vi "FetchRX.vi"(8 "error in (no error)":errorcluster, 11 "reference in":refnum<class "niMmWave_Reciever.lvclass">) -> (0 "error out":errorcluster, 2 "RX burst data":refnum<class "mmWave data.lvclass">, 3 "reference out":refnum<class "niMmWave_Reciever.lvclass">)   [LabVIEW 2019, in "niMmWave_Reciever.lvclass"]
doc: "Fetches RX IQ data from isnturment"
uses:
  niMmWave_Reciever.lvclass
  C:/Barkhausen mmWave radar/Development/modules/mmw_instrument/src_LabVIEW/Host/SubVIs/mmWave instrument_class/mmWave instrument.lvclass
  mmWave data_class/mmWave data.lvclass
  mmWave HW Control/HW custom error.ctl
  mmWave instrument_class/Instrument state.ctl
  IQBurst_memo_class/IQBurst_memo.lvclass
  C:/Barkhausen mmWave radar/Development/modules/mmw_instrument/src_LabVIEW/Host/SubVIs/mmWave data_class/mmWave data.lvclass
  23a7541f-384f-44a9-b270-a12c5ae2c0ad.vi
  <vilib>/addons/Modulation/Analog/MT Resample (Complex Cluster).vi
  <vilib>/addons/Modulation/Analog/support/Validators/mod_Fractional Resample Validate.vi
  <vilib>/addons/Modulation/Analog/support/Validators/mod_Check Flush State.vi
  <vilib>/addons/Modulation/Analog/support/mod_FractionalResampler.vi
  <vilib>/addons/Modulation/Analog/support/mod_Integer Rate Interpolation.vi
  <vilib>/addons/Modulation/Analog/support/mod_Set Error Source.vi
  <vilib>/addons/Modulation/Analog/support/Validators/mod_Validate Complex Waveform.vi
  <vilib>/addons/Modulation/Analog/support/mod_PerformResampling.vi
  <vilib>/addons/Modulation/Analog/support/Validators/mod_WFErrorHandler.vi
  <userlib>/_OpenG.lib/string/string.llb/Trim Whitespace (String)__ogtk.vi
  <vilib>/Utility/error.llb/Error Cluster From Error Code.vi
  <vilib>/addons/Modulation/Analog/support/mod_Resampling Factors.vi
  <vilib>/addons/Modulation/Analog/support/mod_ResamplingFilter.vi
  <vilib>/addons/Modulation/Analog/support/mod_Generate Integer Interpolation Filter.vi
  mmWave HW Control/mmWave HW Control.lvlib
  mmWave instrument_class/mmWave instrument.lvclass
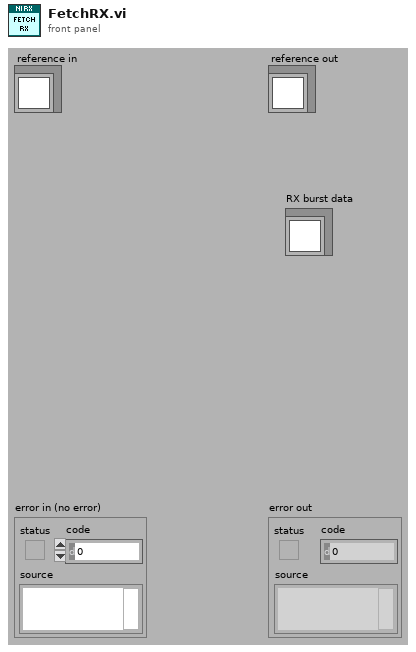
[diagram p1: front panel]
types:
  T1 = typedef "mmWave instrument.lvclass/Instrument state.ctl" = enum16{"Off", "Initialization", "Configuration", "Running", "Calibration"}
  T2 = typedef "mmWave HW Control.lvlib/HW custom error.ctl" = u16
  T3 = typedef "niMmWave_Reciever.lvclass/ObjectAttributesRef.ctl" = refnum<data-value>
  T4 = typedef "niMmWave_Reciever.lvclass/ObjectAttributes.ctl" = cluster{"session":T5[], "HW.RX devices":T19, "RF config":T20, "RX trigger options":T21, "RX samples":i32, "RX Fs":dbl}
  T5 = typedef "Session.ctl" = cluster{"3620 session":refnum<queue>, "tx baseband session":T6, "rx baseband session":T14, "tx gain (dB)":dbl, "rx gain (dB)":dbl, "hardware configuration":T15, "gain ranging":T17[], "pxi trigger bus information":T18}
  T6 = typedef "Tx Baseband Session.ctl" = cluster{"3610 session":T7, "7902 reference":T13}
  T7 = typedef "ni3610_and_ni3630_Driver_Lib.lvlib/Main Settings.ctl" = cluster{"VISA resource name":refnum<visa-resource-name>, "Address Space":T8, "window_offset":u32, "register_addresses":T9, "required_MM_fpga_version":cluster{"signature":u32, "hardware":u32, "current revision":u32, "oldest revision":u32}, "CPLD Oldest Compat Version ":cluster{"hardware":u32, "CPLD firmware":u32}, "MM_FPGA_image_location":string, "is_init":bool, "card_type":T10, "DacLmkConfigFileName":string, "AdcLmkConfigFileName":string, "AdcConfigFileName":string, "DacConfigFileName_RevA":string, "DacConfigFileName_RevB":string, "Mulde hardware revision":u8, "bypass DAC PLL\n":bool, "IQ Card Revision":T11, "board capability":T12}
  T8 = typedef "VISA Register Access Address Space.ctl" = u16
  T9 = typedef "ni3610_and_ni3630_Driver_Lib.lvlib/Register Adresses.ctl" = cluster{"MM based Registers":cluster{"Revision":u32, "OldestCompatRev":u32, "signature":u32, "scratch":u32, "LedControl":u32, "BoardHwRev":u32, "BoardControl":u32, "ThermalStatus":u32, "BasebandStatus":u32, "BasebandControl":u32, "BasebandAuxSetup":u32, "BasebandAuxStatus":u32, "LmkSyncOutSetup":u32, " AdcSyncOutSetup":u32, " InjSyncOutSetup":u32, " PxiTrig0OutSetup":u32, " PxiTrig1OutSetup":u32, " PxiTrig2OutSetup":u32, " PxiTrig3OutSetup":u32, " PxiTrig4OutSetup":u32, " PxiTrig5OutSetup":u32, " PxiTrig6OutSetup":u32, " PxiTrig7OutSetup":u32}, "CPLD based Registers":cluster{"SlaveSignature":u32, "SlaveRevision":u32, "SlaveOldestCompatRev":u32, "SlaveScratch":u32, "SlaveSetup":u32, "SlaveStatus":u32, "IDacReg_offset":u32, "LMKRegGrp0_offset":u32, "QDacReg_offset":u32, "BrdTempSensorVal":u32, "TempSensorPowerDown":u32, "GPIOReg_offset":u32, "IAdcReg_offset":u32, "QAdcReg_offset":u32, "LMKRegGrp1_offset":u32, "QadcTempSensorVal":u32, "IadcTempSensorVal":u32, "RevisionReg":u32, "VcxoReg":u32, "CpldStatusReg":u32, "PowerReg":u32, "VBiasEnReg":u32, "ExtRefOeReg":u32, "QdacCtrlReg":u32, "QdacStatusReg":u32, "IdacCtrlReg":u32, "IdacStatusReg":u32, "QdacJtagIn":u32, "QdacJtagOut":u32, "IdacJtagIn":u32, "IdacJtagOut":u32, "IqDcSetupReg":u32, "QadcStatusReg":u32, "IadcStatusReg":u32, "BrdSetupReg":u32, "IqDcRevisionReg":u32, "PllStatusReg":u32, "EndpointScratchReg":u32, "AdcSyncCfgReg":u32, "IqCardOpampReg":u32}, "CPLD Register Offset":u32, "MM  Register Offset":u32, " PxiTrig0OutSetup":u32}
  T10 = typedef "ni3610_and_ni3630_Driver_Lib.lvlib/Base Card Type.ctl" = enum16{"unspecified", "ADC", "DAC"}
  T11 = typedef "ni3610_and_ni3630_Driver_Lib.lvlib/IQ Card Revision.ctl" = enum16{"RevA", "RevB", "RevC", "RevD"}
  T12 = typedef "ni3610_and_ni3630_Driver_Lib.lvlib/Board Capability.ctl" = cluster{"baseband sync":enum16{"no baseband sync", "baseband sync"}}
  T13 = typedef "Blank FPGA Reference.ctl" = refnum<k20>
  T14 = typedef "Rx Baseband Session.ctl" = cluster{"3630 session":T7, "7902 reference":T13}
  T15 = typedef "Hardware Configuration.ctl" = cluster{"direction":T16, "baseband only":bool}
  T16 = typedef "Direction.ctl" = enum16{"Transceiver", "Receiver", "Transmitter"}
  T17 = typedef "Gain Ranging.ctl" = cluster{"gain ranging active scope":string, "gain ranging stream session":refnum<k20>}
  T18 = typedef "PXI Trigger Bus Info.ctl" = cluster{"chassis resource name":refnum<visa-resource-name>, "7902R (TX)":i16, "3610 (TX)":i16, "3620 (IF)":i16, "3630 (RX)":i16, "7902R (RX)":i16}
  T19 = typedef "mmWave HW Control.lvlib/HW RX resources cluster.ctl" = cluster{"HW.IF":tag, "HW.ADC":refnum<visa-resource-name>, "HW.RX FPGA":tag}
  T20 = typedef "mmWave HW Control.lvlib/HW RX RF config cluster.ctl" = cluster{"Gain":dbl, "Frequency":dbl, "mmWave adapter":string}
  T21 = typedef "TX trigger config.ctl" = cluster{"delay":dbl, "trig source":T22, "PXI src":i32, "export":T23, "PXI dest":i32}
  T22 = typedef "FPGA Utility.lvlib/FPGA driver trigger source.ctl" = enum16{"Use Tclk", "PXI_Trig", "Aurora RX trig"}
  T23 = typedef "FPGA Utility.lvlib/FPGA driver trigger destination.ctl" = enum16{"None", "Source trig", "Synced trig", "Delayed sync"}
  T24 = typedef "Constants.ctl" = cluster{"data clock rate (Hz)":dbl, "sample rate (Hz)":dbl, "sample rate selector string":string, "default tx bitfile path":path, "default rx bitfile path":path, "default proc bitfile path":path}
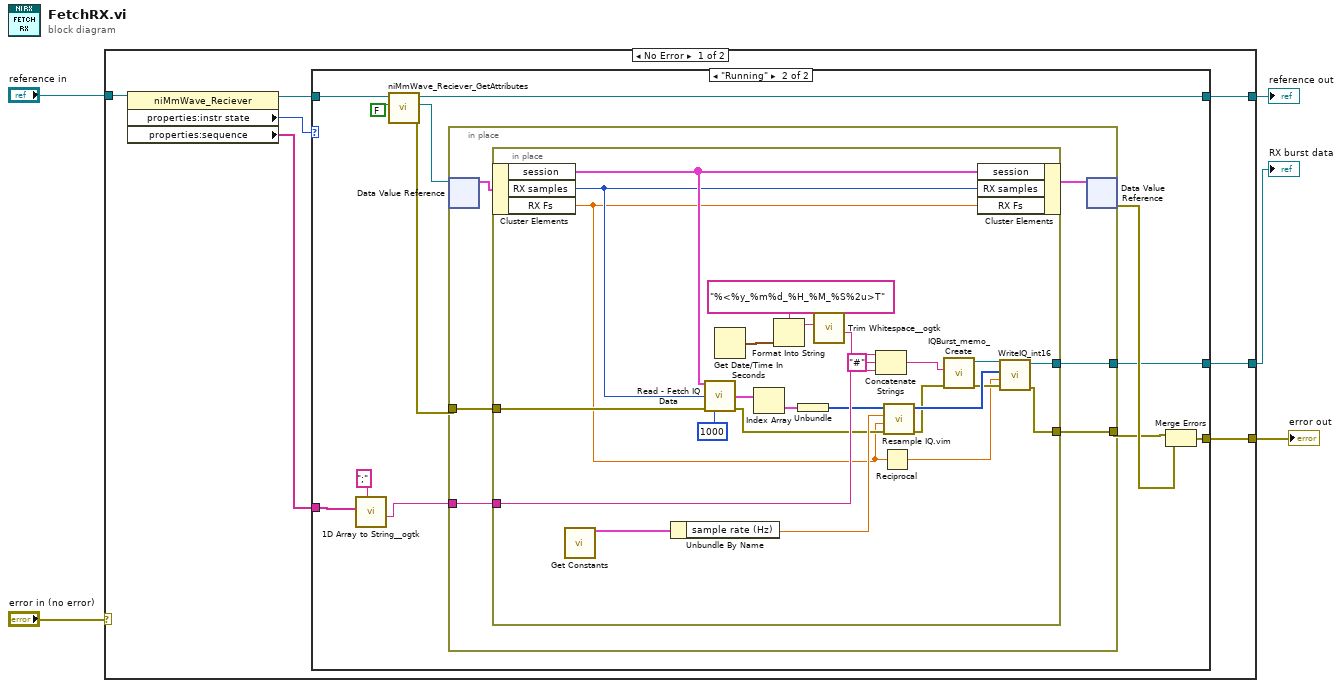
[diagram p0: block diagram]
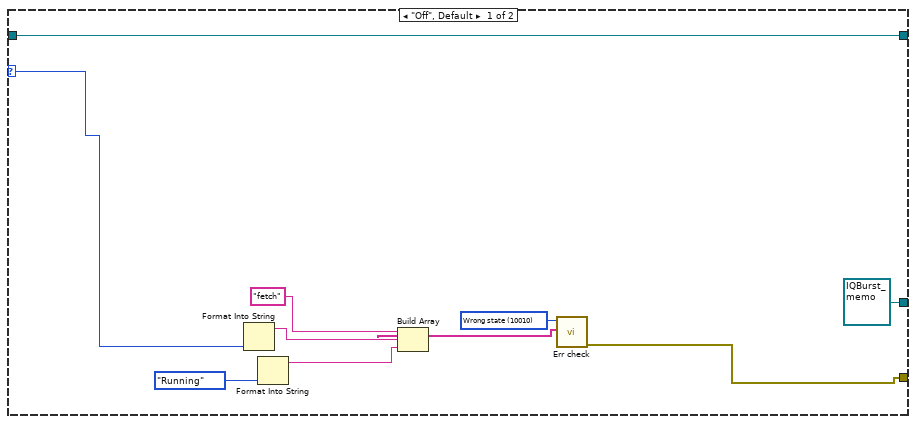
[diagram p2: hidden frame]
diagram:
  n1 = case shown="No Error" "error in (no error)" {
    selector: "error in (no error)" -> [_ w67]
    tunnel: [w12 w67] -> w4
    tunnel: [w11 w66] -> w2
    tunnel: "reference in" -> [w10 w66]
    tunnel: [w6 _] -> w1
    frame No Error {
      n2 = property class="niMmWave_Reciever"(reference=w10) -> (reference out=w9:refnum<class "niMmWave_Reciever.lvclass">, "properties:instr state"=w8:T1, "properties:sequence"=w7:string[])  [unwired: 1 in, 1 out]
      n3 = case shown="\"Running\"" w8 {
        selector: w8 -> [w15 _]
        tunnel: [w14 w34] -> w12
        tunnel: [w22 w31] -> w11
        tunnel: w9 -> [w22 w29]
        tunnel: w7 -> [_ w24]
        tunnel: [refnum<class "IQBurst_memo.lvclass"> refnum ("reference out") w27] -> w6
        frame "Off", Default {
          w21 = T2 10010 items=["TX list"=10000, "TX length"=10001, "RX length"=10002, "Fs"=10003, "RF Fc"=10004, "Wrong state"=10010] ("HW custom err")
          n4 = Format Into String(w15) -> (resulting string=w19:string)  [unwired: 3 in, 1 out]
          n5 = Format Into String(Instrument_state."Running" ("properties:instr state")) -> (resulting string=w16:string)  [unwired: 3 in, 1 out]
          n6 = Build Array("fetch", w19, w16) -> (w18:string[])
          n7 = call "Err check.vi"("Variant Control"=w18, "HW custom err"=w21) -> ("error out"=w14:errorcluster)  [unwired: 9 in]
        }
        frame "Running" {
          n8 = call <userlib>:"1D Array to String__ogtk.vi"("delimiter (Tab)"=";", "Array of Strings"=w24) -> ("delimited string"=w23:string)  [unwired: 9 in]
          n9 = call "niMmWave_Reciever_GetAttributes.vi"("return data? (T)"=FALSE, "reference in"=w29) -> ("error out"=w28:errorcluster, "attributes ref"=w30:T3, "reference out"=w31:refnum<class "niMmWave_Reciever.lvclass">)  [unwired: 6 in, 1 out]
          n10 = in-place {
            in-place-border: w28 -> [w38]
            in-place-border: w23 -> [w37]
            in-place-border: [w36] -> w27
            in-place-border: [w35] -> w26
            n11 = in-place-dvr #1(w30) -> (w39:T4)  [unwired: 1 out]
            n12 = in-place {
              in-place-border: w38 -> [w63]
              in-place-border: w37 -> [w54]
              in-place-border: [w51] -> w36
              in-place-border: [w43] -> w35
              n13 = in-place-cluster #2(w39) -> ("session"=w64:T5[], "RX samples"=w50:i32, "RX Fs"=w42:dbl)
              n14 = call "Get Constants.vi"() -> ("constants"=w57:T24)  [unwired: 15 in]
              n15 = Unbundle By Name(w57) -> ("sample rate (Hz)"=w47:dbl)
              n16 = call "Read - Fetch IQ Data.vi"("session in"=w64, "number of samples"=w50, "error in"=w63, "Timeout (ms)"=1000) -> ("data [channel]"=w62:cluster{"data":i16[]}[], "error out"=w46:errorcluster)  [unwired: 9 in, 1 out]
              n17 = Get Date/Time In Seconds() -> (seconds since 1Jan1904=w60:timestamp)
              n18 = Index Array(array=w62) -> (element=w61:cluster{"data":i16[]})  [unwired: 1 in]
              n19 = Format Into String(format string="%<%y_%m%d_%H_%M_%S%2u>T", w60) -> (resulting string=w58:string)  [unwired: 2 in, 1 out]
              n20 = Unbundle(w61) -> ("data"=w49:i16[])
              n21 = call-poly <userlib>:"Trim Whitespace__ogtk.vi"("String in"=w58) -> ("String out"=w56:string)  [unwired: 6 in]
              n22 = Concatenate Strings(w56, "#" ("string"), w54) -> (w53:string)
              n23 = Reciprocal(x=w42) -> (1/x=w41:dbl)
              n24 = call "Resample IQ.vim"("error in (no error)"=w46, "FS out"=w42, "Fs in"=w47, "data in"=w49) -> ("error out"=w45:errorcluster, "resampled data"=w48:i16[])  [unwired: 6 in]
              n25 = call "IQBurst_memo_Create.vi"("error in (no error)"=w45, "burst name"=w53) -> ("error out"=w44:errorcluster, "reference out"=w52:refnum<class "IQBurst_memo.lvclass">)  [unwired: 8 in]
              n26 = in-place-cluster #2("session"=w64, "RX samples"=w50, "RX Fs"=w42) -> (w40:T4)
              n27 = call-dynamic "WriteIQ_int16.vi"("error in (no error)"=w44, "dt"=w41, "data"=w48, "reference in"=w52) -> ("error out"=w43:errorcluster, "reference out"=w51:refnum<class "IQBurst_memo.lvclass">)  [unwired: 6 in]
            }
            n28 = in-place-dvr #1(w40) -> (w33:errorcluster)  [unwired: 1 out]
          }
          n29 = Merge Errors(w26, w33) -> (w34:errorcluster)
        }
      }
    }
    frame Error {
    }
  }
  "error out" <- w4
  "reference out" <- w2
  "RX burst data" <- w1
